vi "RetoWhile.vi"() -> ()   [LabVIEW 2022 SP3]
panel:
  out "No. Iteraciones":i32
  in  "Ingresa un número hasta el que quieras que cuente, papi":i32
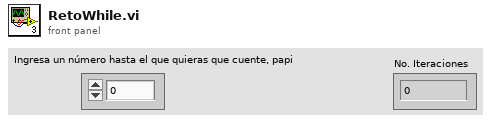
[diagram p1: front panel]
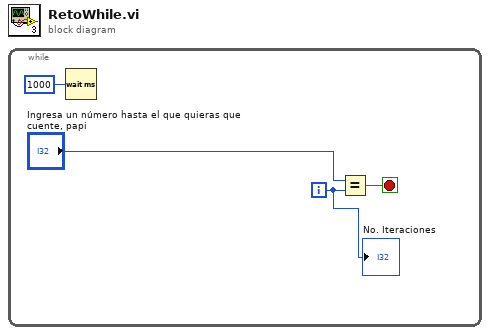
[diagram p0: block diagram]
diagram:
  n1 = while {
    i -> [w1]
    stop <- w2 stop-if-true
    n2 = Wait (ms)(milliseconds to wait=u32 1000) -> ()  [unwired: 1 out]
    n3 = Equal?(x="Ingresa un número hasta el que quieras que cuente, papi", y=w1) -> (x = y?=w2:bool)
    "No. Iteraciones" <- w1
  }
